vi "TestMotor.vi"() -> ()   [LabVIEW 2018]
panel:
  in  "Percent Open":dbl min=0.0 max=100.0 step=0.5
  out "Zaber Motor Error":errorcluster
  in  "stop":bool
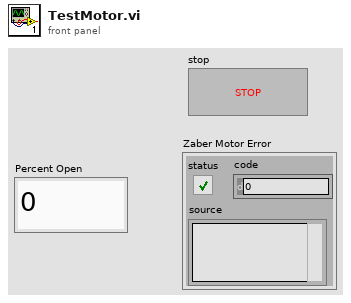
[diagram p1: front panel]
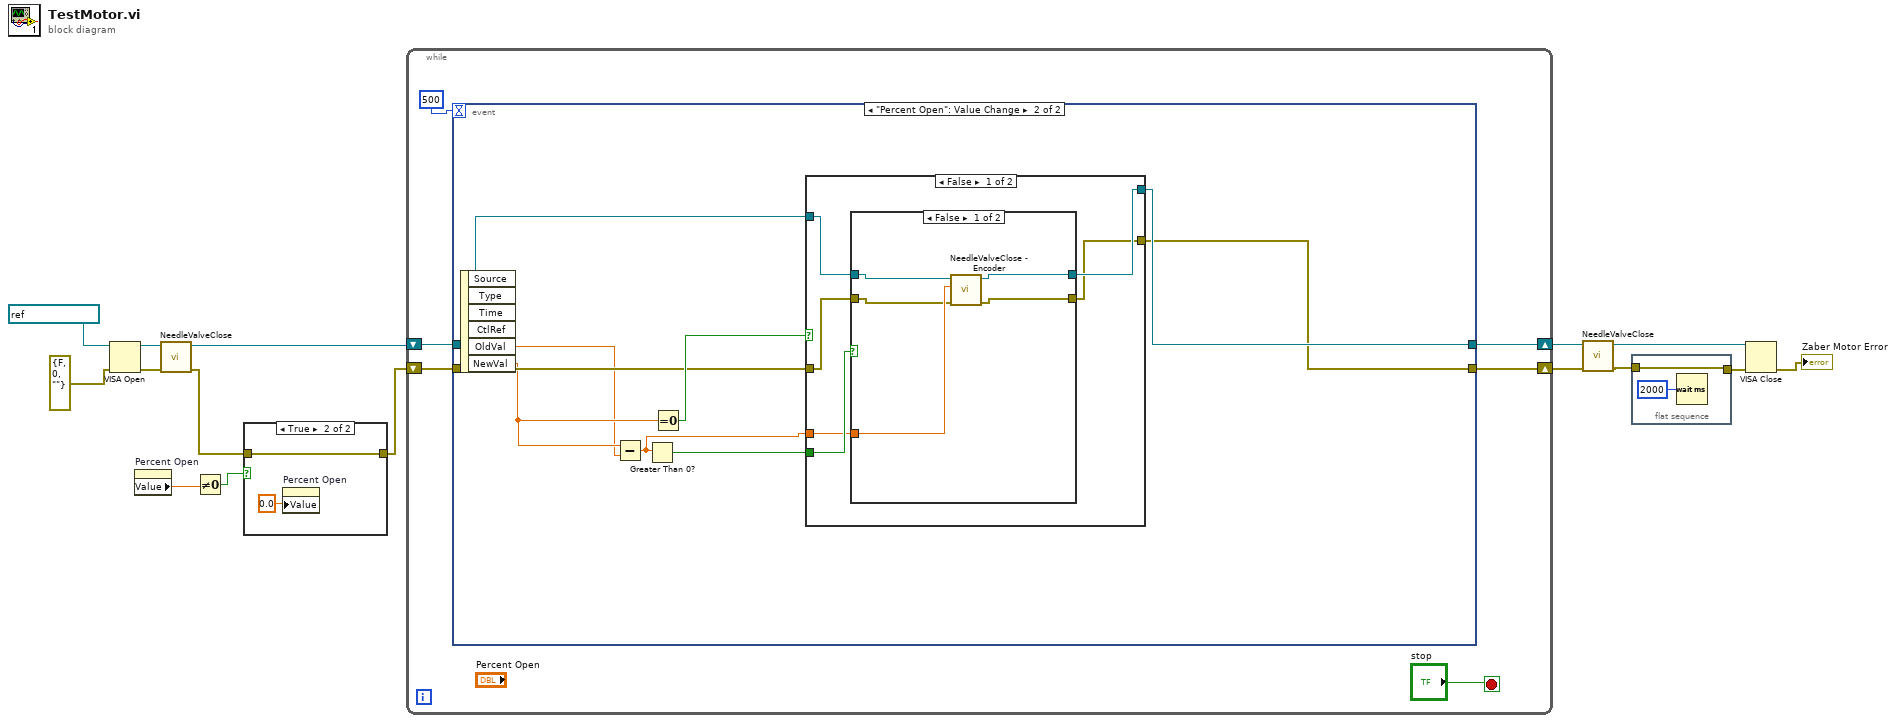
[diagram p0: block diagram]
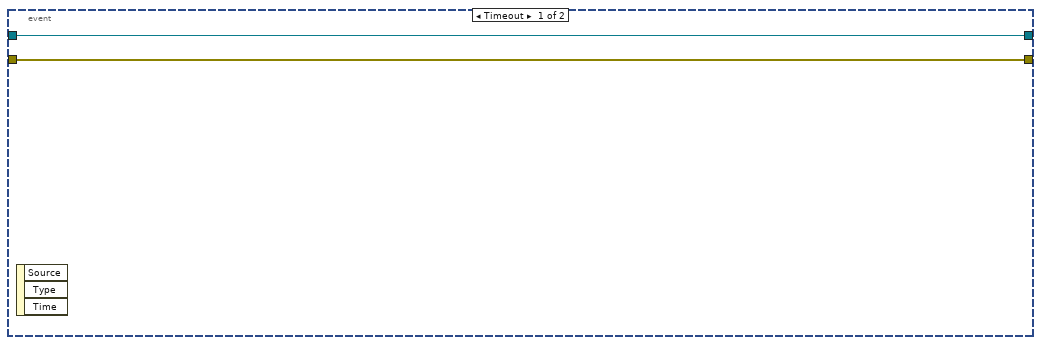
[diagram p3: hidden frame]
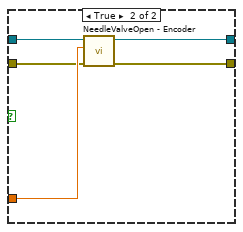
[diagram p4: hidden frame]
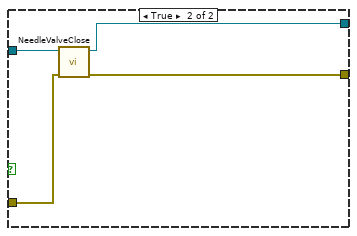
[diagram p5: hidden frame]
diagram:
  n1 = VISA Open(error in (no error)=errorcluster {"status"=FALSE, "code"=0, "source"=""}, VISA resource name=refnum<visa-resource-name> "ZaberMotor") -> (VISA resource name=w13:refnum<visa-resource-name>, error out=w12:errorcluster)  [unwired: 3 in]
  n2 = property on="Percent Open" class="DigNum (strict)"() -> ("Value"=w4:dbl)  [unwired: 2 in, 2 out]
  n3 = call "NeedleValveClose.vi"("error in (no error)"=w12, "VISA resource name"=w13) -> ("error out"=w2:errorcluster, "VISA resource name out"=w5:refnum<visa-resource-name>)  [unwired: 8 in]
  n4 = Not Equal To 0?(x=w4) -> (x != 0?=w3:bool)
  n5 = case shown="True" w3 {
    tunnel: w2 -> [w16 w18]
    tunnel: [w16 w18] -> w1
    frame False {
    }
    frame True {
      n6 = property on="Percent Open" class="DigNum (strict)"("Value"=0.0 ("Percent Open")) -> ()  [unwired: 2 in, 2 out]
    }
  }
  n7 = while {
    shift-right: [w19] -> w7
    shift-left: w5 -> [w22]
    shift-right: [w20] -> w6
    shift-left: w1 -> [w21]
    stop <- "stop" stop-if-true
    n8 = event shown="[1] \"Percent Open\": Value Change" {
      selector: _ -> [_ _]
      dyn-events: _ -> [_ _]
      timeout: 500 -> [_ _]
      tunnel: w22 -> [w25 w32]
      tunnel: w21 -> [w26 w31]
      tunnel: [w26 w29] -> w20
      tunnel: [w25 w30] -> w19
      event Timeout {
        n9 = event-data() -> ()  [unwired: 1 in, 3 out]
      }
      event "Percent Open": Value Change {
        n10 = event-data() -> ("OldVal"=w27:dbl, "NewVal"=w28:dbl)  [unwired: 1 in, 4 out]
        n11 = Subtract(x=w28, y=w27) -> (x-y=w33:dbl)
        n12 = Greater Than 0?(x=w33) -> (x > 0?=w34:bool)
        n13 = Equal To 0?(x=w28) -> (x = 0?=w35:bool)
        n14 = case shown="False" w35 {
          tunnel: [w40 w55] -> w30
          tunnel: [w39 w54] -> w29
          tunnel: w34 -> [w41 _]
          tunnel: w33 -> [w38 _]
          tunnel: w32 -> [w36 w53]
          tunnel: w31 -> [w37 w52]
          frame False {
            n15 = case shown="False" w41 {
              tunnel: [w46 w51] -> w40
              tunnel: [w45 w50] -> w39
              tunnel: w38 -> [w44 w49]
              tunnel: w37 -> [w42 w48]
              tunnel: w36 -> [w43 w47]
              frame False {
                n16 = call "NeedleValveClose - Encoder.vi"("error in (no error)"=w42, "Percent Difference"=w44, "VISA resource name"=w43) -> ("error out"=w45:errorcluster, "VISA resource name out"=w46:refnum<visa-resource-name>)  [unwired: 7 in]
              }
              frame True {
                n17 = call "NeedleValveOpen - Encoder.vi"("error in (no error)"=w48, "Percent Difference"=w49, "VISA resource name"=w47) -> ("error out"=w50:errorcluster, "VISA resource name out"=w51:refnum<visa-resource-name>)  [unwired: 7 in]
              }
            }
          }
          frame True {
            n18 = call "NeedleValveClose.vi"("error in (no error)"=w52, "VISA resource name"=w53) -> ("error out"=w54:errorcluster, "VISA resource name out"=w55:refnum<visa-resource-name>)  [unwired: 8 in]
          }
        }
      }
    }
  }
  n19 = call "NeedleValveClose.vi"("error in (no error)"=w6, "VISA resource name"=w7) -> ("error out"=w9:errorcluster, "VISA resource name out"=w10:refnum<visa-resource-name>)  [unwired: 8 in]
  n20 = flat-sequence {
    tunnel: w9 -> [w56]
    tunnel: [w56] -> w8
    frame #0 {
      n21 = Wait (ms)(milliseconds to wait=u32 2000) -> ()  [unwired: 1 out]
    }
  }
  n22 = VISA Close(VISA resource name=w10, error in (no error)=w8) -> (error out=→"Zaber Motor Error":errorcluster)
